vi "test_ClientFGV_GetClientTwice_ClientOnlyCreatedOnce.vi"(8 "error in":errorcluster) -> (0 "error out":errorcluster, 2 "result":string, 3 "pass":bool)   [LabVIEW 2020, in "MeasurementServerTests.lvlib" / "gRPC Utilities Tests.lvlib"]
uses:
  gRPC Utilities Tests.lvlib
  Runtime/MeasurementLink gRPC Utilities/TypeDefs/Client Pool FGV Action.ctl
  Fake Client Action.ctl
  Runtime/MeasurementLink gRPC Utilities/MeasurementLink gRPC Utilities.lvlib
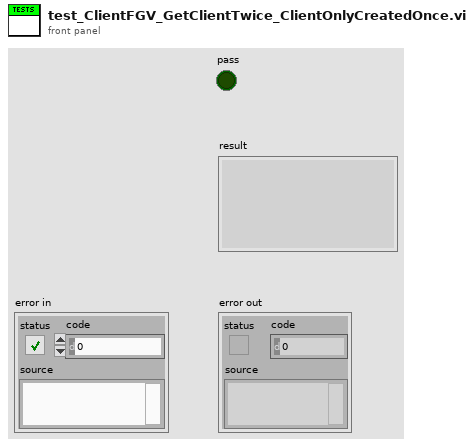
[diagram p1: front panel]
types:
  T1 = typedef "MeasurementServerTests.lvlib/gRPC Utilities Tests.lvlib/Fake Client Action.ctl" = enum16{"Generate New Id", "Reset", "Error on Next Call"}
  T2 = typedef "MeasurementLink gRPC Utilities.lvlib/Client Pool FGV Action.ctl" = enum16{"Get Client", "Recreate Client"}
  T3 = typedef "grpc-lvsupport-release.lvlib/grpcId.ctl" = u64
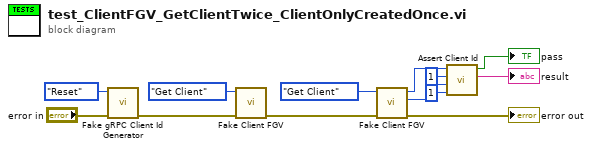
[diagram p0: block diagram]
diagram:
  n1 = call "Fake gRPC Client Id Generator.vi"("error in"="error in", "action"=Fake_Client_Action."Reset") -> ("error out"=w8:errorcluster)  [unwired: 8 in, 1 out]
  n2 = call "Fake Client FGV.vi"("error in"=w8, "action"=Client_Pool_FGV_Action."Get Client") -> ("error out"=w10:errorcluster)  [unwired: 7 in, 2 out]
  n3 = call "Fake Client FGV.vi"("error in"=w10, "action"=Client_Pool_FGV_Action."Get Client") -> ("error out"=→"error out":errorcluster, "unique id out"=w5:u64, "grpc client id"=w6:T3)  [unwired: 7 in]
  n4 = call "Assert Client Id.vi"("expected unique id"=u64 1, "actual unique id"=w5, "expected client id"=u64 1, "actual client id"=w6) -> ("result"=→"result":string, "pass"=→"pass":bool)  [unwired: 6 in]
